vi "Dequeue Message.vi"(8 "error in (no error)":errorcluster, 11 "OOQMH in":refnum<class "OOQMH.lvclass">) -> (0 "error out":errorcluster, 2 "Message out":refnum<class "Message.lvclass">, 3 "OOQMH out":refnum<class "OOQMH.lvclass">)   [LabVIEW 2024, in "OOQMH.lvlib" / "OOQMH.lvclass"]
uses:
  OOQMH.lvclass
  Message/Message.lvclass
  OOQMH.lvclass/OOQMH.ctl
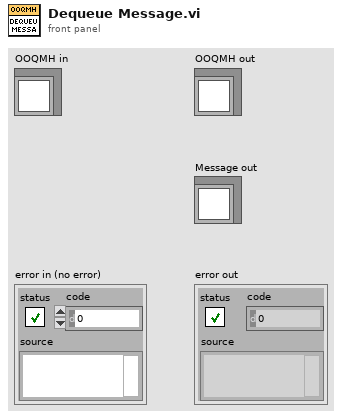
[diagram p1: front panel]
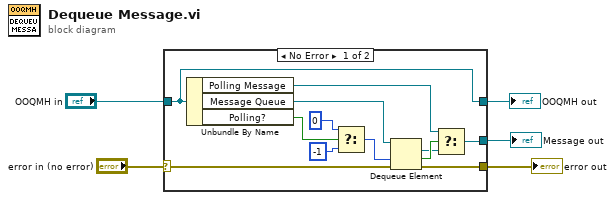
[diagram p0: block diagram]
diagram:
  n1 = case shown="No Error" "error in (no error)" {
    selector: "error in (no error)" -> [w15 w19]
    tunnel: [w14 w19] -> w4
    tunnel: [w17 w18] -> w2
    tunnel: "OOQMH in" -> [w17 w18]
    tunnel: [w6 _] -> w1
    frame No Error {
      n2 = Unbundle By Name(w17) -> ("Polling Message"=w7:refnum<class "Message.lvclass">, "Message Queue"=w16:refnum<queue>, "Polling?"=w13:bool)
      n3 = Select(t=0, s=w13, f=-1) -> (s? t:f=w10:i32)
      n4 = Dequeue Element(queue=w16, timeout in ms (-1)=w10, error in (no error)=w15) -> (element=w8:refnum<class "Message.lvclass">, timed out?=w9:bool, error out=w14:errorcluster)  [unwired: 1 out]
      n5 = Select(t=w7, s=w9, f=w8) -> (s? t:f=w6:refnum<class "Message.lvclass">)
    }
    frame Error {
    }
  }
  "error out" <- w4
  "OOQMH out" <- w2
  "Message out" <- w1
